vi "2025_day11_Task01.vi"() -> ()   [LabVIEW 2025]
uses:
  <userlib>/_OpenG.lib/string/string.llb/openg_string.lvlib
panel:
  out "Task 1 (# of valid paths)":i32
  in  "Switch":bool caption="Ex. Data  vs.  User Data"
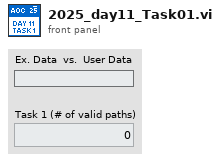
[diagram p1: front panel]
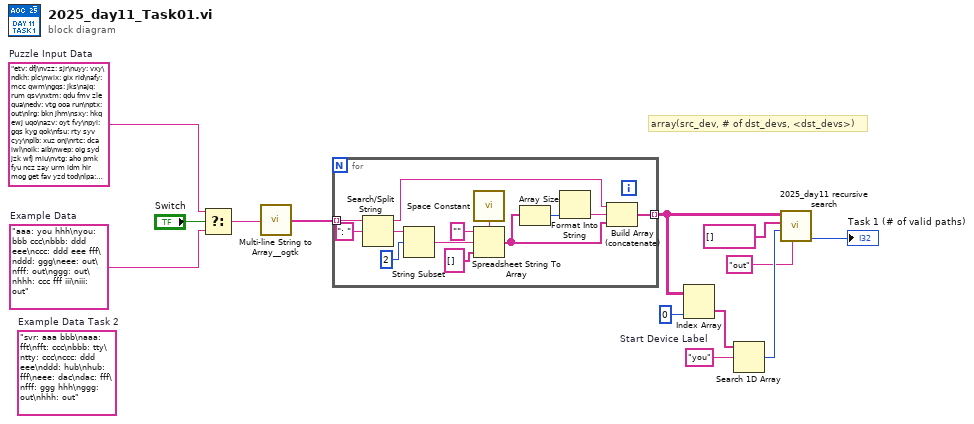
[diagram p0: block diagram]
diagram:
  w8 = "you"  # Start Device Label
  (unwired) "svr: aaa bbb\naaa: fft\nfft: ccc\nbbb: tty\ntty: ccc\nccc: ddd eee\nddd: hub\nhub: fff\neee: dac\ndac: fff\nfff: ggg hhh\nggg: out\nhhh: out"  # Example Data Task 2
  w12 = "etv: dfj\nvzz: sjr\nuyy: vxy\ndkh: plc\nwix: gix rid\nafy: mcc qwm\ngqs: jks\najq: rum qsv\nxtm: qdu fmv zle qua\nedv: vtg ooa run\nptx: out\nlrg: bkn jhm\nsxy: hkq ewj uqo\nazv: oyt fvy\npyi: gqs kyg qok\nfsu: rty syv cyy\nplb: xuz onj\nrtc: dca iwl\noik: aib\nwep: oig syd jzk wfj miu\nvtg: aho pmk fyu ncz zay urm idm hir mog get fav yzd tod\nlpa: qrk vtf\nbld: giq tsm\ndap: buc\nmrs: izf mig upb\njgz: zlm lub\nowr: ldt mmh atk hbl\nxck: aon dxx qil\namo: xcr mii bjo vih\nqrk: gew plm\nqwm: jts jfm slu\njef: pln ekw kev gct bdn mbk aok owg oko\nzfc: uof tnc cvp umv\naok: vsp ipu\nwyi: lva wcy ehz cww\nxlp: wxd uhm\nent: kdt iyl\nnps: out\nlbf: fct jgv fjv\nxdw: wyi dkh lkl gej\nzen: btr azo\nocw: ewg dje\ncyr: gtn jft rgu\nopc: lva wcy ehz\nllq: wqs fye\nwqp: hur zve gme bsq\ncyy: kel\nyvq: sqt eyl\nwbn: run ooa vtg\ntrr: cvp\njgn: xdw enq kgm\ndbv: zpe dac prb\nmcv: fta\nkyr: rum qsv gqx\nbqm: enq kgm xdw\nocx: out\ntzd: pvb\nfcx: dca\nonj: tam krr\nhbf: kgm xdw kel\ntam: enq\nucu: bxd bpp uhm wxd\nanb: rmq azo btr\numv: tzd sjn lyt pyi tkr fmn fzq gys lej lue nds pfb vsn tly\nnrk: tzi ovs fie\nfqm: iwl dca\nkxc: mxc buc\ngnf: vmg\nvrt: uof tnc umv cvp\nsth: tcy uyy kyi jni\nzoy: tse vnq\ncvp: lyt pyi tkr tzd sjn tyz dbv jlv pfb lfp vsn lag tly cag gys lej llq lue fzq fmn\ncjd: izf\ndsh: pzd pkp\nzwo: you\nrip: zve bsq gme egx\nlzm: nps tvp\niyl: fte eyn\nehf: hpu dmh tyj\nldt: zsl edv bye\nceu: aib nyd\nwzs: tnc uof cvp\nisj: you\nshe: bzz\nezy: dxz\nuoy: zlv dje kuz\nftc: uof\nruq: run syn vtg\nqil: yju abb cga\nwfj: uof umv cvp\nrfg: uoy\nnix: you dca\njmk: dsh clr\nmbk: ydl kma\nvxn: cyr\njlv: dap cso cfg\nkma: gwy yqe sjr\nsyv: kel xpi enq\njur: onj ywl\nxrv: tnc uof umv\nxuz: wjy\ngxq: uxl zpb\nfwo: gxq jic\nwzp: uof tnc\nmmw: pln qbi sod vld fia ekw bdn gct pnu qmb lsh ynt kez gqp mbk nzi owg rna ypn\niev: aon aro\nfja: out\npyh: xdw\nbza: ooa run\npgq: rgo vli\nvsn: kyg gqs qok xyv\nkev: ipu\nwra: ygj qan wix\nowg: rps ixy jtm\nafd: meb smh fxy\nyys: ajq vvu jft gtn\nbsq: jpz kyr\nnwj: bgb fvy bvx oyt\nvih: yni oik tmb\nxzr: ooa syn vtg\ngme: kyr jpz gmr\nffx: pnu lsh nvi qmb pln wjg fia ypn oko rna nzi\nsjr: kel xpi enq kgm xdw\nsof: xdw kgm kel\nooa: xmx pmk cfa jmk arx aho ybp ncz fyu urm mog hir zay afd amo ipk gwv tod ssw yzd wdo get\nfek: mkm rys msy rfg\nygj: gix rid jjq\nqdv: pff vol yys kvu\nmbn: pff yys vol kvu\nnvi: dse uyr drp yib\nabb: jpb zwo rtc oru\ncfg: dtm buc qvu mxc fcx\nheo: csx\ndfj: qwm\nhpu: dga\nxfj: qdu fmv\nkvu: vvu\nqvu: iwl you\nyqe: xpi xdw kel\nohw: ydf ftc trr ice\nuza: out\nfhr: gew ozc plm yin\njks: iwl dca\nyci: vli\nbxd: anb sqs zen\nzpg: pwi biy oxs\nlhe: jhm\nzve: gmr\ndxz: you dca iwl\nzlv: yww xzr\nbye: syn run\nlbs: run\nmeb: oxh\ngvs: pbf vkz kdl zpm xjc\nctg: rys mkm rfg\nuzl: gxq ppc ftd\nkyc: aro qil dxx\ntgd: out\nipu: vtf fhr\nxcf: kax rmq\nrgu: rum\nwcy: mbn vxn exo\njtm: gqb hns\nmsy: ocw\nfta: msq opj pyh\nqqp: pnt\nfhs: sof vnq bqm\nfkr: ooa run syn\noru: iwl\nzay: ohw uwi ylt\nfbw: gxq ftd\ngkz: efh rjf ehf\nypn: ksm dse\nsmh: mbi\nzod: tjc syv gur\nclr: ekx pzd pkp\nsal: bqm sof tse vnq\nbiy: msq\nydo: mzz lks\ngwy: xpi enq\niul: wxd bpp uhm dpl\nxtr: vtg syn\nirs: aoy jfc gkz\nnpo: ecc plc\nrgo: zoy ozf dlw sal\nhkq: ovs tgd\nrmq: ruq pmf\nbry: fsu vfl\nrbj: tnc\nydl: hbf yqe nur gwy\npwi: xod zad\nlog: wix ygj\npet: bry\nayv: gkz jfc\nmlw: eyn fqb\nfpz: ldt mmh\ndse: mcv\ndac: fsr dxz\nwjy: enq xpi kgm xdw\nubn: xuz iiu ywl\nqsv: ctg xlp iul sfr owr ucu she jbu rpd his qqe log wra ike qnq\nqip: run syn\nyag: tcy jni kyi uyy\neyn: hkq uqo\nyco: yvq ehs pds\nftd: zpb uxl\nhvx: out\ntle: you\nfyu: bte gvs duj\nvkz: rbj\nzsl: vtg\nrsm: izf mig upb\ntyj: vmg\noig: cvp umv\nsod: rso ydl vzz\ntek: mko dfj\niiu: wjy tam krr\ngix: kdj xaf wbn\ndtm: dca iwl\nrhp: rkt wkx ent\ncom: you\naho: gvs kpp\ntap: mrs zux rsm\ngew: tid\nske: qiv\nivz: vtg syn run\nxjc: vrt rbj xrv ciz\nbig: qsv rum\ndzc: kel xdw enq xpi kgm\nvxy: syn vtg run ooa\nyka: kcq\nojj: xfj\nfhw: run ooa syn\nnns: wkx rkt\nazo: itn pmf\nslu: big qcc\nozw: tnc umv\ncww: mbn vxn qdv\nrpd: qns xlj bzz\nrjf: lup dmh hpu\nfia: rps dss pet jtm\nfav: kpp gvs\nice: uof\nsjn: bxq fye\njhm: vpv\nkcg: jfc\nasr: eyn sxy fte\noxh: jgz xpc\nwls: nps\ndss: xmj\nnpb: out\ngiq: pds yvq\nqbi: kma xqv\nybp: meb\nxod: enq kgm kel\npmk: xbg uwi ylt ohw\natk: zsl edv lbs\nbqw: tvp tcs\nzxl: out\njfm: qcc\nepx: xpi enq kgm kel\nmiu: tnc umv\nmig: qsv rum\nksm: mjd\nkif: out\newg: fhw\naao: gix\nsyn: yzd ipk pmk xmx ybp arx afd\nvqs: bkn\necx: bkn jhm\nkui: tvp\nxxk: ztv owl\nmsq: xpi xdw\novs: out\nfte: ewj uqo\nfie: out\ntjr: hnn ymb csx mne\nciz: cvp umv uof\nvtt: lub zlm\nkbi: khv vli\nidm: xcr bjo mii\nztv: tjr adc kvg\nbjo: yni lmp\nsqs: kax btr azo\nnds: kyc\ntod: mii\nvli: dlw ozf sal fhs zoy\njfc: efh\nfzq: xck\nwuz: kyi uyy tcy\nwjg: ipu vsp\nsyd: cvp tnc\nbvx: you iwl\nuqo: tss fie\necc: zux rsm yrg cjd\nyzd: wse tjg\nlub: uof umv cvp\nwdo: bjo\nkax: itn pmf\nxaf: syn\ntcy: qip fkr ivz euw\ncuq: out\nxej: afy\nojr: gxq ppc\nxmj: zod\nqnq: wix\nplm: epx jgn dzc yzf\noko: jur plb ubn\ncpb: lzm wls kui bqw\naro: abb\nyqa: bvx\ncuw: out\njzi: ovc jgv fjv fct\ncso: qvu buc\nuxl: cpb cua hpo\nrps: xmj gqb hns bry\ndhu: cpb\nrty: kel enq xdw\npkp: wzs ozw rdz\nyin: dzc jgn epx\ndmh: ael vmg\ntjg: lks mzz jiw\narx: ydo wse\nznz: vqs ecx\ngmr: rum qsv\noka: che lhe\nlfp: kxc cso dap\ntcs: out\nynm: rum gqx\nlsh: vzz\nyzf: xdw kgm xpi kel\nvee: sai ent\nmxc: iwl\nopj: xdw kgm xpi enq\nrso: hbf sjr yqe nur\nhbl: zsl\nbtr: itn ruq\nbuc: you dca iwl\nbbd: cuq ptx\nymb: rin\nfxy: oxh hph mbi\nssw: cmp tjg wse\neyl: xzt aih ske\nplc: mrs zux rsm cjd yrg\nlmq: tsm yco\npmf: vtg ooa\nmkm: uoy ocw\nhir: fxy lmh\nmko: mcc fft\nxzt: jpt qiv npb\nglm: flh lva\ntid: xpi enq xdw\nkvg: hnn\nduj: pbf kdl zpm vkz\nfye: ege meg nwj\nflh: qdv\nfap: biy dwu pwi\nmmh: bye edv\nbxq: ege yqa\nyml: out\nzad: xpi kel\nozf: vnq\nkbt: yag\neqz: rfg rys\nevp: rgo khv vli\nvsp: qrk fhr\nuwi: zfc ftc trr\nhis: aao ygj\nfvy: iwl\nncz: ohw uwi agx xbg\ngej: wcy flh\nadc: csx mne ymb hnn\npzd: rdz ozw wzs\ncsx: bbd rin xli\nxyv: fqm\nbjw: rgo\ncmp: mzz lks\nwyc: xfj ghv\nmog: gvs duj\nqok: fqm zob jks nix\njni: ivz qip\njbu: qns\nipk: gvs duj bte\nooi: cuw zxl vpv\noxs: xod pyh opj msq\njpb: you iwl\nhur: jpz\npyd: out\nxli: ptx yml uza\nkdt: sxy fte\nqpq: ztv kcq\nfqb: nrk\nlyt: pvb cfg cso\nowl: yva heo tjr adc\nqan: rid gix\nlag: bxq\ntse: enq xpi kel\nzux: upb mig\nqet: ywl\nyww: run syn vtg\nenq: dkh lkl wyc jvl rip etv tek twe xej wqp wyi opc gej ojj glm\ngys: dac prb\ncua: fnn kui wls bqw\nyju: oru rtc com jpb\nlva: mbn exo\nqiv: out\njiw: umv cvp uof\ngqc: big\nyni: aib nyd\njvl: xfj xtm ghv\ngur: xdw xpi enq kgm kel\nxbg: trr zfc\njts: big\nfwa: fjv jgv ovc qqp\nhns: zod fsu\nlej: zpe prb ezy\ndga: fja\nycs: ehs\nzpb: cpb hpo\njpz: rum qsv\nexo: vol kvu\nkel: twe sjk gej npo xrh glm wyc lkl rip\novc: znz pnt\nqcc: rum qsv\ntnc: jlv dbv tyz sjn tzd pyi fzq lue nds llq lej gys cag lag vsn lfp pfb\npnt: vqs lrg ecx\nupb: gqx\nkdj: syn ooa\npds: sqt lkn\njzk: umv uof\nxlj: sth wuz\ngqp: dss\nfmv: gqx rum qsv\nyva: mne csx\nvnq: xdw xpi kgm kel\nizf: gqx rum\nrna: ubn qet\nsfr: mmh ldt hbl\nhph: ozy xpc vtt\ncga: zwo com\nbpp: zen sqs anb xcf\nvol: rgu\nkyg: zob fqm jks nix\nche: ooi bkn\ndpl: sqs anb\nget: xcr\ncfa: clr iua\nvld: ubn jur qet\nqdu: qsv gqx\nafz: sai ent wkx\nbdn: dse uyr drp\nlue: xck rdy\nefh: gnf lup tyj\ngtn: gqx\npln: pgq\nbte: vkz kdl\njnv: cua cpb hpo\nppc: dhu jnv uxl\nlmh: oxh\nmjd: pwi oxs dwu\negx: jpz\nekx: wzs rdz\nydf: umv tnc\nvmg: fja meh\npvb: fcx buc dtm\nylt: ydf trr zfc ice\nujj: wxd uhm bpp bxd dpl\nktf: wix aao\nvbp: qns kbt bzz xlj\nkgm: wqp opc gej ojj npo glm xrh lkl wyc rip xej\nghv: qua zle\nrun: ncz fyu pmk cfa xmx ybp arx aho jmk tod ssw ipk gwv fav get wdo zay mog hir idm urm amo afd\nyib: zpg mcv mjd\nuof: tly lag vsn lfp lue nds llq gys lej cag fzq fmn tkr pyi sjn tzd dbv jlv\nixy: hns\newj: tss tzi ovs fie\neuw: syn run ooa\nxqv: nur hbf yqe\nfft: slu jts sqf\nwqs: azv meg ege nwj\nkuz: flj xzr xtr yww fhw\nmeh: out\ntly: iev xck\nvpv: out\nzpe: isj ava\nwxd: xcf\ncag: xyv gqs qok\nsvr: ffx jef mmw\npff: vvu gtn jft\ngct: lpa ipu\nxia: ztv\nmkk: aoy jfc\nbkn: vpv kif cuw\nagx: ftc ice\nmii: ceu\nlkn: xzt aih ske\nhnn: rin bbd\nczr: bzz xlj\nkhv: ozf dlw fhs zoy\nozy: lub\nmbi: xpc vtt ddt ozy jgz\nlmp: wep\nxrh: ecc plc tap\nyrg: upb\nwwm: hbo yco tsm giq ycs\nzlm: tnc uof\nwse: lks mzz\ntsm: pds\nrid: kdj xaf wbn\nehs: sqt\njjq: wbn bza xaf\nsjk: egx bsq gme zve\ngqb: zod fsu\nprb: isj fsr\njgv: znz oka\nkrr: kel xpi enq xdw\nflj: ooa vtg syn\nrdy: aro aon\nuhm: sqs\nnzi: lpa\nael: meh hvx\ntzi: out\nnyd: wfj miu jzk syd oig\nrin: pyd uza\nvvu: rum qsv\nkpp: zpm xjc vkz\naon: yju\naih: jpt\nurm: fxy\nkez: kma xqv\nnur: kel xdw enq\nfmn: ezy zpe\nrkt: kdt iyl asr\nzpm: rbj ciz\ntss: out\nzob: iwl dca you\npfb: cso cfg pvb dap\nhbo: ehs\ngqx: fpz owr iul wra log qqe eqz rpd ike ujj\nxpi: etv rip jvl lkl wyc dkh xrh tek xej glm npo gej ojj sjk wyi wqp opc\njft: rum qsv gqx\npbf: vrt ciz\ntvp: out\nbgb: iwl\nlup: ael vmg dga\nsqt: ske\nlks: umv cvp uof\npnu: kbi yci evp pgq\ndxx: cga\noyt: dca iwl\nrum: ujj ike fek eqz qqe his rpd ktf ucu fpz czr owr sfr vbp ctg xlp\nqua: rum\nozc: jgn\ntjc: kgm\nqns: yag sth\njpt: out\ngwv: clr dsh\ndca: yka fbw nns jzi irs uzl kcg ojr lmq rhp afz fwo lbf xxk xia wwm bld mkk qpq ayv\nmcc: jts gqc\niwl: jzi kxt nns fwa uzl irs lmq afz xia xxk lbf vee ayv qpq bld\nehz: exo vxn mbn\ndlw: tse sof\nitn: syn ooa run\nfjv: znz\nqqe: rys sqo\nzle: gqx rum\nike: wxd bpp bxd dpl\nkyi: fkr\nvtf: ozc gew\nava: iwl\nfct: oka znz pnt\nhpo: wls kui bqw fnn\nxmx: dsh iua\nlkl: mko\nvfl: syv rty gur\nwkx: kdt iyl\nrys: mby ocw\ntmb: wep nyd aib\nsqo: uoy ocw\nbzz: wuz\nmby: ewg zlv\nxcr: yni oik ceu tmb lmp\njic: dhu jnv uxl zpb\naoy: rjf ehf\ntyz: iev\nmzz: tnc umv cvp\nrdz: uof tnc\nxpc: lub zlm\nuyr: zpg mcv fap\nmne: bbd xli\nkxt: sai\nekw: pgq evp bjw\nsqf: ynm big\ndrp: mjd zpg fap\nmeg: tle oyt bvx bgb fvy\nfsr: dca\ndwu: opj zad xod pyh\nddt: wzp\ntkr: dac prb ezy\nyou: nns ojr rhp yka fwa xxk xia wwm kcg\ndje: flj\nkdl: rbj vrt xrv ciz\nfnn: ocx\nkcq: kvg yva tjr adc\nynt: pet dss rps\naib: syd jzk miu\nqmb: ubn\nege: fvy bgb tle\nsai: mlw\ntwe: afy mko dfj\niua: pzd pkp\nywl: krr tam"  # Puzzle Input Data
  w1 = "aaa: you hhh\nyou: bbb ccc\nbbb: ddd eee\nccc: ddd eee fff\nddd: ggg\neee: out\nfff: out\nggg: out\nhhh: ccc fff iii\niii: out"  # Example Data
  # "array(src_dev, # of dst_devs, <dst_devs>)"
  n1 = Select(t=w12, s="Switch", f=w1) -> (s? t:f=w11:string)
  n2 = call <userlib>:"Multi-line String to Array__ogtk.vi"("string"=w11) -> ("lines"=w10:string[])
  n3 = for {
    tunnel: w10 -> [w26] mode=indexing
    tunnel: [w15] -> w6 mode=indexing
    n4 = Search/Split String(string=w26, search string/char (-)=": ") -> (substring before match=w14:string, match + rest of string=w24:string)  [unwired: 1 in, 1 out]
    n5 = String Subset(string=w24, offset (0)=2) -> (substring=w22:string)  [unwired: 1 in]
    n6 = call <vilib>:"Space Constant.vi"() -> ("String"=w21:string)
    n7 = Spreadsheet String To Array(delimiter (Tab)=w21, format string="", spreadsheet string=w22, array type (2D Dbl)=string[] []) -> (array=w16:string[])
    n8 = Array Size(array=w16) -> (size(s)=w18:i32)
    n9 = Format Into String(w18) -> (resulting string=w17:string)  [unwired: 3 in, 1 out]
    n10 = Build Array (concatenate)(w14, w17, w16) -> (w15:string[])
  }
  n11 = Index Array(array=w6, index (col)=0 ("disabled index (col)")) -> (element=w4:string[])  [unwired: 1 in]
  n12 = Search 1D Array(1D array=w4, element=w8) -> (index of element=w9:i32)  [unwired: 1 in]
  n13 = call "2025_day11 recursive search.vi"("End Device Label"="out", "Dev idx"=w9, "path history in"=string[] [], "Data in"=w6) -> ("# of valid paths out"=→"Task 1 (# of valid paths)":i32)  [unwired: 5 in, 2 out]
